vi "franch_error_detect.vi"(4 "error in (no error)":errorcluster, 6 "key bit sequence":u8[](array[numeric]), 7 "input bit sequence":u8[](array[numeric])) -> (0 "error out":errorcluster, 3 "bit-error rate":dbl)   [LabVIEW 2012]
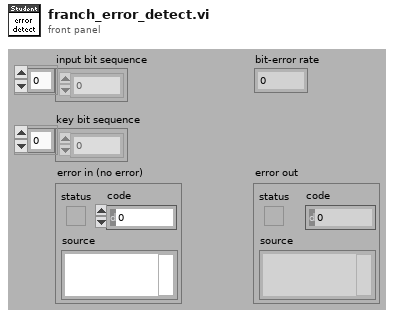
[diagram p1: front panel]
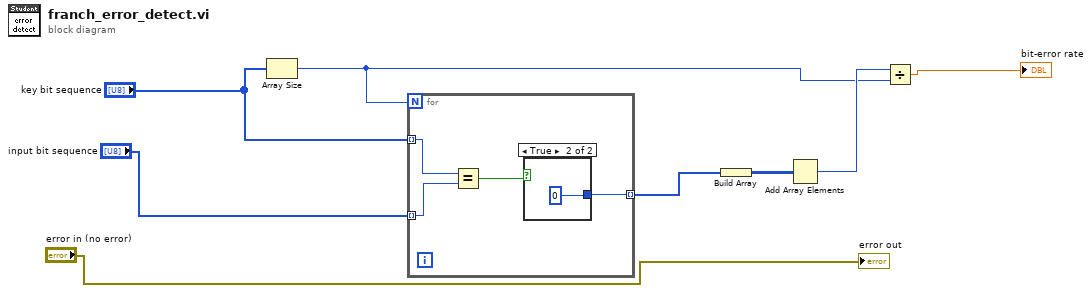
[diagram p0: block diagram]
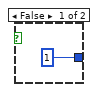
[diagram p2: hidden frame]
diagram:
  n1 = Array Size(array="key bit sequence") -> (size(s)=w5:i32)
  n2 = for {
    N: w5 -> [_]
    tunnel: "key bit sequence" -> [w12] mode=indexing
    tunnel: "input bit sequence" -> [w11] mode=indexing
    tunnel: [w9] -> w7 mode=indexing
    n3 = Equal?(x=w12, y=w11) -> (x = y?=w10:bool)
    n4 = case shown="True" w10 {
      tunnel: [1 0] -> w9
      frame False {
      }
      frame True {
      }
    }
  }
  n5 = Build Array(w7) -> (w8:i32[][])
  n6 = Add Array Elements(numeric array=w8) -> (sum=w6:i32)
  n7 = Divide(x=w6, y=w5) -> (x/y=→"bit-error rate":dbl)
  "error out" <- "error in (no error)"
